vi "run_simulation_or_interrupt.vi"(4 "Interrupted?":refnum<vi>, 5 "Specifications":string, 6 "Interrupt Run":refnum<vi>, 7 "Output File Loaded?":refnum<vi>, 10 "Done?":refnum<vi>, 11 "Run":refnum<vi>) -> (0 "OK?":bool, 1 "standard output":string, 2 "standard error":string, 3 "TMP Filepath":path)   [LabVIEW 2019]
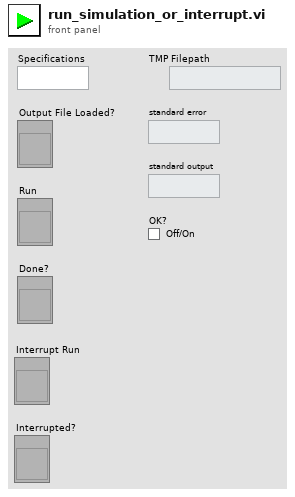
[diagram p1: front panel]
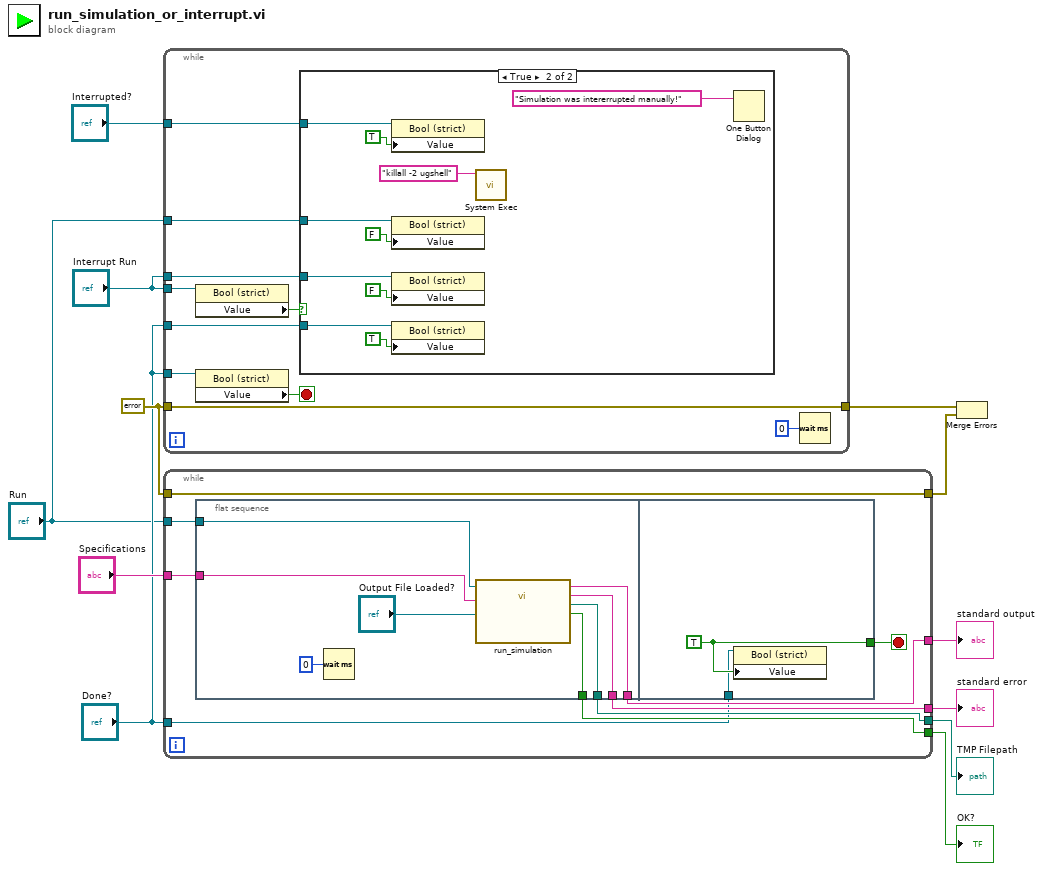
[diagram p0: block diagram]
diagram:
  w7 = errorcluster {"status"=FALSE, "code"=0, "source"=""} ("error constant")
  n1 = while {
    tunnel: w7 -> [w22]
    tunnel: [w22] -> w5
    tunnel: "Done?" -> [w18]
    tunnel: "Run" -> [w17]
    tunnel: "Interrupt Run" -> [w16]
    tunnel: "Interrupted?" -> [w15]
    tunnel: "Done?" -> [w14]
    tunnel: "Interrupt Run" -> [w13]
    stop <- w20 stop-if-true
    n2 = property class="Bool (strict)"(reference=w13) -> ("Value"=w19:bool)  [unwired: 1 in, 2 out]
    n3 = property on="Property Node" class="Bool (strict)"(reference=w14) -> ("Value"=w20:bool)  [unwired: 1 in, 2 out]
    n4 = case shown="True" w19 {
      tunnel: w18 -> [_ w26]
      tunnel: w17 -> [_ w25]
      tunnel: w16 -> [_ w24]
      tunnel: w15 -> [_ w23]
      frame False {
      }
      frame True {
        n5 = property on="Property Node" class="Bool (strict)"(reference=w23, "Value"=TRUE ("Interrupted")) -> ()  [unwired: 1 in, 2 out]
        n6 = property on="Property Node" class="Bool (strict)"(reference=w25, "Value"=FALSE ("Run")) -> ()  [unwired: 1 in, 2 out]
        n7 = property on="Property Node" class="Bool (strict)"(reference=w24, "Value"=FALSE ("Interrupt Run")) -> ()  [unwired: 1 in, 2 out]
        n8 = property on="Property Node" class="Bool (strict)"(reference=w26, "Value"=TRUE ("Done")) -> ()  [unwired: 1 in, 2 out]
        n9 = call <vilib>:"System Exec.vi"("command line"="killall -2 ugshell") -> ()  [unwired: 7 in, 4 out]
        n10 = One Button Dialog(message="Simulation was intererrupted manually!") -> ()  [unwired: 1 in, 1 out]
      }
    }
    n11 = Wait (ms)(milliseconds to wait=u32 0) -> ()  [unwired: 1 out]
  }
  n12 = while {
    tunnel: w7 -> [w41]
    tunnel: [w41] -> w6
    tunnel: "Specifications" -> [w40]
    tunnel: [w39] -> w9
    tunnel: [w38] -> w10
    tunnel: [w36] -> w11
    tunnel: [w35] -> w12
    tunnel: "Done?" -> [w34]
    tunnel: "Run" -> [w33]
    stop <- w37 stop-if-true
    n13 = flat-sequence {
      tunnel: w40 -> [w48]
      tunnel: [w46] -> w39
      tunnel: [w45] -> w38
      tunnel: [w44] -> w36
      tunnel: [w43] -> w35
      tunnel: w33 -> [w42]
      tunnel: [w51] -> w37
      tunnel: w34 -> [w50]
      frame #0 {
        n14 = Wait (ms)(milliseconds to wait=u32 0) -> ()  [unwired: 1 out]
        n15 = call "run_simulation.vi"("Output File Loaded?"="Output File Loaded?", "inputSpecs"=w48, "Run"=w42) -> ("OK?"=w46:bool, "TMP Filepath"=w45:path, "standard error"=w43:string, "standard output"=w44:string)  [unwired: 5 in]
      }
      frame #1 {
        w51 = TRUE ("Done")
        n16 = property on="Property Node" class="Bool (strict)"(reference=w50, "Value"=w51) -> ()  [unwired: 1 in, 2 out]
      }
    }
  }
  "standard error" <- w12
  "standard output" <- w11
  "TMP Filepath" <- w10
  "OK?" <- w9
  n17 = Merge Errors(w5, w6) -> ()  [unwired: 1 out]
